vi "DAQmx Create Channel (CI-Pulse Ticks).vi"(0 "task in":refnum<k21>, 1 "maximum value":dbl=1000000.0 format="%.6f", 2 "minimum value":dbl=1000.0 format="%.6f", 5 "counter":tag, 7 "name to assign":string, 9 "source of ticks":tag="OnboardClock", 11 "error in":errorcluster) -> (4 "task out":refnum<k21>, 15 "error out":errorcluster)   [LabVIEW 2020]
doc: "Creates a channel to measure pulse specifications, returning the measurements as pairs of high ticks and low ticks. With the exception of devices that support multi-counter tasks, you can create only one counter input channel at a time with this VI because a task can contain only one counter input channel. To read from multiple counters simultaneously, use a separate task for each counter. Connect the input signal to the default input terminal of the counter unless you select a different input terminal."
uses:
  nilvaiu.dll
panel:
  # "input limits"
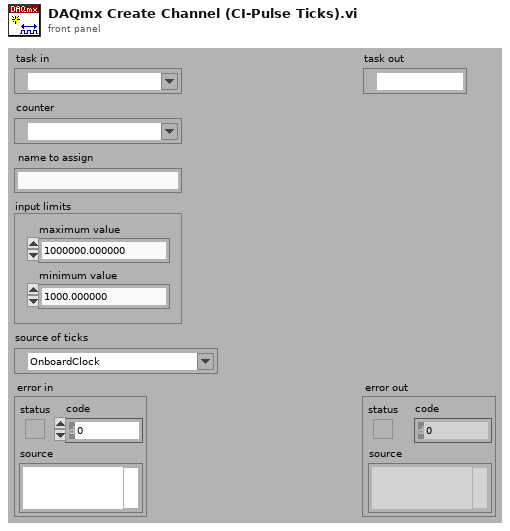
[diagram p1: front panel]
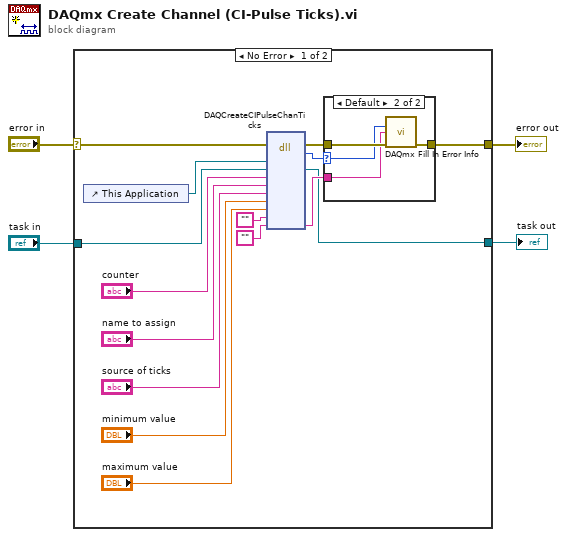
[diagram p0: block diagram]
diagram:
  n1 = case shown="No Error" "error in" {
    selector: "error in" -> [w6 w26]
    tunnel: [w10 w26] -> w4
    tunnel: [w8 w25] -> w3
    tunnel: "task in" -> [w7 w25]
    frame No Error {
      n2 = control-ref of="This Application"() -> (w16:refnum<vi>)
      n3 = dll-call lib="nilvaiu.*" fn="DAQCreateCIPulseChanTicks"(error in=w6, "lvAppRef"=w16, "refObjPtr"=w7, "counter"="counter", "channelNameIn"="name to assign", "sourceTerminal"="source of ticks", "minVal"="minimum value", "maxVal"="maximum value", "channelNamesOut"="", "extendedErrorInfo"="") -> (error out=w19:errorcluster, "return type"=w18:i32, "refObjPtr"=w8:refnum<k21>, "extendedErrorInfo"=w17:string)  [unwired: 9 in, 1 out]
      n4 = case shown="Default" w18 {
        selector: w18 -> [_ w22]
        tunnel: w19 -> [w20 w24]
        tunnel: [w20 w23] -> w10
        tunnel: w17 -> [_ w21]
        frame 0 {
        }
        frame Default {
          n5 = call "DAQmx Fill In Error Info.vi"("status code"=w22, "extended error info"=w21, "error in"=w24) -> ("error out"=w23:errorcluster)  [unwired: 1 in, 11 out]
        }
      }
    }
    frame Error {
    }
  }
  "error out" <- w4
  "task out" <- w3
